vi "Day 06 (Part Two).vi"() -> ()   [LabVIEW 2021]
panel:
  out "result":u64
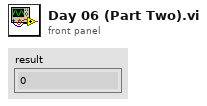
[diagram p1: front panel]
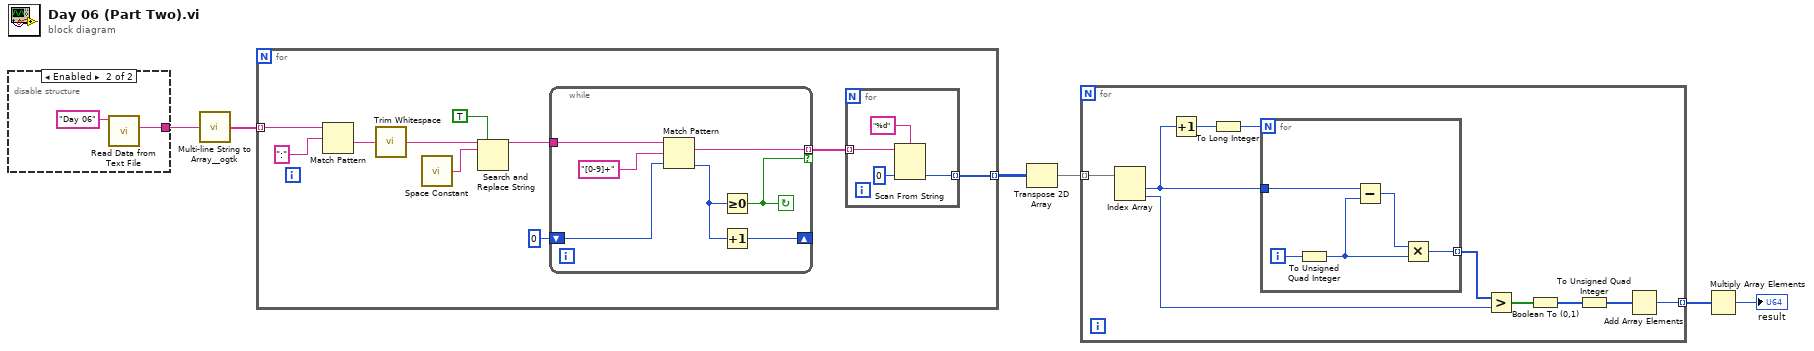
[diagram p0: block diagram]
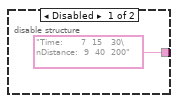
[diagram p2: hidden frame]
diagram:
  n1 = disable-structure shown="Enabled" {
    disable-tunnel: ["Time:      7  15   30\nDistance:  9  40  200" w9] -> w6
    frame Disabled {
    }
    frame Enabled {
      n2 = call "Read Data from Text File.vi"("Subfolder"="Day 06") -> ("data"=w9:string)  [unwired: 10 in]
    }
  }
  n3 = call <userlib>:"Multi-line String to Array__ogtk.vi"("string"=w6) -> ("lines"=w5:string[])
  n4 = for {
    tunnel: w5 -> [w19] mode=indexing
    tunnel: [w15] -> w4 mode=indexing
    n5 = Match Pattern(string=w19, regular expression=":") -> (after substring=w17:string)  [unwired: 1 in, 3 out]
    n6 = call <vilib>:"Trim Whitespace.vi"("string"=w17) -> ("trimmed string"=w12:string)  [unwired: 1 in]
    n7 = call <vilib>:"Space Constant.vi"() -> ("String"=w11:string)
    n8 = Search and Replace String(replace all?=TRUE ("replace all? (F)"), input string=w12, search string=w11) -> (result string=w13:string)  [unwired: 5 in, 3 out]
    n9 = while {
      tunnel: w13 -> [w30]
      shift-right: [w28] -> _
      shift-left: 0 -> [w27]
      tunnel: [w24] -> w14 mode=indexing if=w25
      stop <- w25 continue-if-true
      n10 = Match Pattern(string=w30, regular expression="[0-9]+", offset (0)=w27) -> (match substring=w24:string, offset past match=w26:i32)  [unwired: 2 out]
      n11 = Greater Or Equal To 0?(x=w26) -> (x >= 0?=w25:bool)
      n12 = Increment(x=w26) -> (x+1=w28:i32)
    }
    n13 = for {
      tunnel: [w22] -> w15 mode=indexing
      tunnel: w14 -> [w21] mode=indexing
      n14 = Scan From String(format string="%d", input string=w21, default 1=u64 0 ("default value 1")) -> (output 1=w22:u64)  [unwired: 2 in, 3 out]
    }
  }
  n15 = Transpose 2D Array(2D array=w4) -> (transposed array=w3:u64[][])
  n16 = for {
    tunnel: w3 -> [w40] mode=indexing
    tunnel: [w34] -> w1 mode=indexing
    n17 = Index Array(array=w40) -> (element #1=w38:u64, element #2=w31:u64)  [unwired: 2 in]
    n18 = Increment(x=w38) -> (x+1=w39:u64)
    n19 = To Long Integer(number=w39) -> (32bit integer=w32:i32)
    n20 = for {
      N: w32 -> [_]
      tunnel: [w43] -> w37 mode=indexing
      tunnel: w38 -> [w41]
      i -> [w44]
      n21 = To Unsigned Quad Integer(1:w44) -> (0:w42:u64)
      n22 = Subtract(x=w41, y=w42) -> (x-y=w45:u64)
      n23 = Multiply(x=w45, y=w42) -> (x*y=w43:u64)
    }
    n24 = Greater?(x=w37, y=w31) -> (0:w36:bool[])
    n25 = Boolean To (0,1)(Boolean=w36) -> (0, 1=w35:i16[])
    n26 = To Unsigned Quad Integer(1:w35) -> (0:w33:u64[])
    n27 = Add Array Elements(numeric array=w33) -> (sum=w34:u64)
  }
  n28 = Multiply Array Elements(1:w1) -> (0:→"result":u64)
